vi "Get List of Synced FPGAs.vi"(8 "error in (no error)":errorcluster, 11 "Tamer in":refnum<class "Tamer.lvclass">) -> (0 "error out":errorcluster, 2 "Synced FPGAs":string[](array[string]), 3 "Tamer out":refnum<class "Tamer.lvclass">)   [LabVIEW 2020, in "Tamer.lvlib" / "Tamer.lvclass"]
uses:
  Tamer.lvclass
  Tamer.lvclass/Tamer.ctl
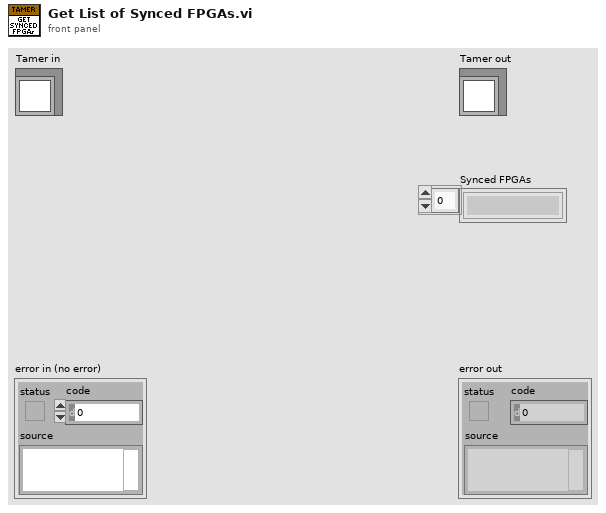
[diagram p1: front panel]
types:
  T1 = typedef "Run Utilities.lvlib/Synchronize FPGA Cluster.ctl" = cluster{"Status":bool, "FPGA Name":string}
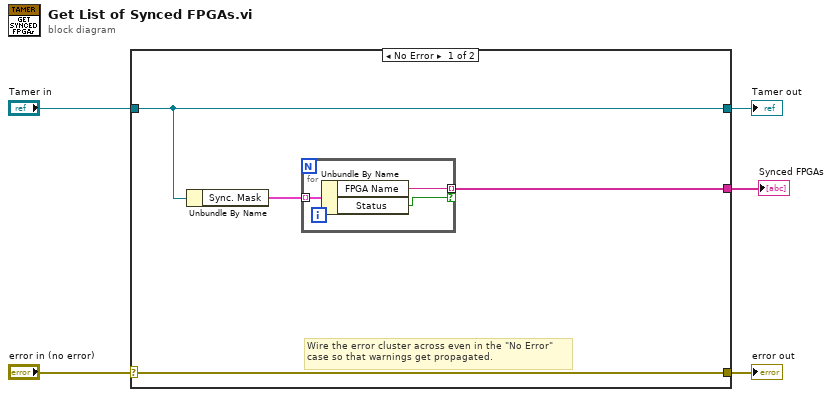
[diagram p0: block diagram]
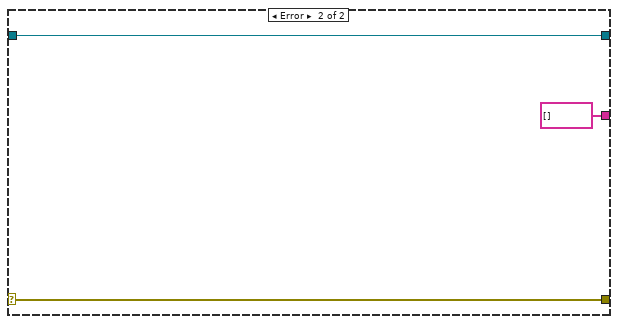
[diagram p2: hidden frame]
diagram:
  n1 = case shown="No Error" "error in (no error)" {
    selector: "error in (no error)" -> [w9 w15]
    tunnel: [w9 w15] -> w4
    tunnel: [w8 w14] -> w2
    tunnel: "Tamer in" -> [w8 w14]
    tunnel: [w6 string[] []] -> w1
    frame No Error {
      # "Wire the error cluster across even in the \"No Error\"\ncase so that warnings get propagated."
      n2 = Unbundle By Name(w8) -> ("Sync. Mask"=w7:T1[])
      n3 = for {
        tunnel: w7 -> [w12] mode=indexing
        tunnel: [w11] -> w6 mode=indexing if=w10
        n4 = Unbundle By Name(w12) -> ("FPGA Name"=w11:string, "Status"=w10:bool)
      }
    }
    frame Error {
    }
  }
  "error out" <- w4
  "Tamer out" <- w2
  "Synced FPGAs" <- w1
